vi "Quick Start.vi"() -> ()   [LabVIEW 2020]
uses:
  <vilib>/Utility/sysdir.llb/System Directory Type.ctl
  Source/Type Defs/Debug Level.ctl
  Source/Sinks/File Sink/File Sink.lvclass
  C:/Users/hughe_cx/Documents/05_repos/LVLog/Source/Sinks/Sink/Sink.lvclass
  Source/LV Log.lvlib
  Source/Logger/Logger.lvclass
panel:
  in  "error in (no error)":errorcluster
  out "error out":errorcluster
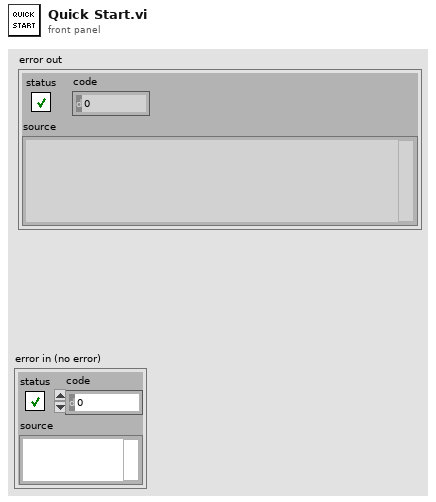
[diagram p1: front panel]
types:
  T1 = typedef "LV Log.lvlib/Debug Level.ctl" = enum16{"DEFAULT", "DEBUG", "INFO", "WARN", "ERROR", "FATAL"}
  T2 = typedef "System Directory Type.ctl" = i32
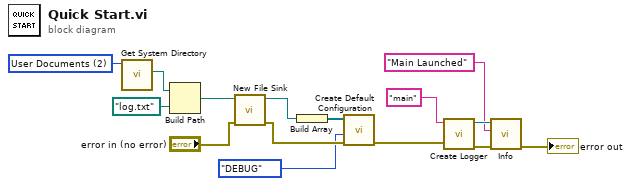
[diagram p0: block diagram]
diagram:
  w9 = T2 2 items=["User Home"=0, "User Desktop"=1, "User Documents"=2, "User Application Data"=3, "User Preferences"=4, "User Temporary"=5, "Public Documents"=6, "Public Application Data"=7, "Public Preferences"=8, "Public Cache"=13, "System Core Libraries"=9, "System Installed Libraries"=10, "Application Files"=11, "Boot Volume Root"=12] ("system directory type")
  n1 = call <vilib>:"Get System Directory.vi"("system directory type"=w9) -> ("system directory"=w8:path)  [unwired: 10 in]
  n2 = Build Path(base path=w8, name or relative path=path "log.txt") -> (appended path=w6:path)
  n3 = call "New File Sink.vi"("error in (no error)"="error in (no error)", "File Path"=w6) -> ("error out"=w2:errorcluster, "File Sink out"=w4:refnum<class "File Sink.lvclass">)  [unwired: 8 in]
  n4 = Build Array(w4) -> (w5:refnum<class "File Sink.lvclass">[])
  n5 = call "Create Default Configuration.vi"("Sinks"=w5, "Debug Level in"=Debug_Level."DEBUG", "error in (no error)"=w2) -> ("error out"=w7:errorcluster)  [unwired: 7 in]
  n6 = call "Create Logger.vi"("error in (no error)"=w7, "Name"="main") -> ("error out"=w14:errorcluster, "Logger out"=w13:refnum<class "Logger.lvclass">)  [unwired: 8 in]
  n7 = call "Info.vi"("error in (no error)"=w14, "Log Text"="Main Launched", "Logger in"=w13) -> ("error out"=→"error out":errorcluster)  [unwired: 6 in, 2 out]
